vi "WPI_CameraCleanup On First Call.vi"(11 "Camera Registry":T1[](array[typedef])) -> ()   [LabVIEW 2017]
doc: "This software is licensed. Open the labview\\readme\\WPI Robotics Library Open Source License.txt file for more information."
uses:
  <vilib>/Rock Robotics/WPI/Camera/WPI_CameraRegistry.ctl
  <vilib>/Rock Robotics/WPI/Camera/WPI_CameraDevRef.ctl
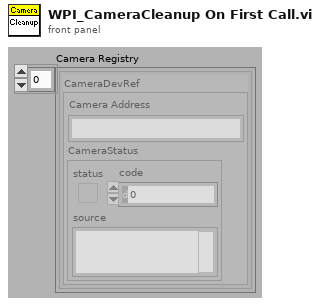
[diagram p1: front panel]
types:
  T1 = typedef "WPI_CameraRegistry.ctl" = cluster{"CameraDevRef":T2}
  T2 = typedef "WPI_CameraDevRef.ctl" = cluster{"Camera Address":string, "CameraStatus":errorcluster}
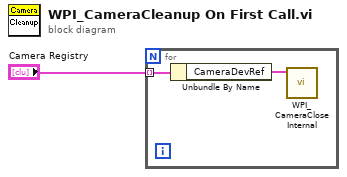
[diagram p0: block diagram]
diagram:
  n1 = for {
    tunnel: "Camera Registry" -> [w3] mode=indexing
    n2 = Unbundle By Name(w3) -> ("CameraDevRef"=w2:T2)
    n3 = call <vilib>:"WPI_CameraClose Internal.vi"("CameraDevRef"=w2) -> ()  [unwired: 2 in, 9 out]
  }
